vi "SS2 Live_Exit Cleanup.vi"(11 "SS2 Live Internal Variables":T1={"okCFrontPanelDevices Refnum"=refnum, "Device Refnum"=refnum, "Display Image"=refnum, "# Live Images"=0, "relative s"=0.0, "# Image Sets"=0, "Message"="", "Current Image Set"=0, "# Datasets"=0, "Current Dataset"=0, "Live Mode"=FALSE, "Recording Mode"=FALSE, "Record Button"=refnum, "Live Button"=refnum, "SS2 Live Gate Data Q Name"="", "Discard First Image"=FALSE, "Image Information"={"Save ROI Only"=FALSE, "Left"=0, "Top"=0, "Right"=0, "Bottom"=0, "Use Current ROI"=FALSE}, "Image Binning Options"={"Use Image Binning"=FALSE, "X Bin"=0, "Y Bin"=0}, "FPGA Serial Number"="", "PCB Version"=enum."PCB 1"} {"Image Binning Options"."Y Bin" min=1; "Image Binning Options"."X Bin" min=1}) -> ()   [LabVIEW 2019]
uses:
  SS2 Live Internal Variables.ctl
  C:/UCLA Thinkpad Google Drive/LabVIEW 2019 SP1/builds/SS2 Live Distribution/Opal Kelly/C# Wrapper/libFrontPanel-csharp.dll
  Opal Kelly/C# Wrapper/libFrontPanel-csharp.dll
  <vilib>/vision/Image Controls.llb/IMAQ Image.ctl
  SS2 Live_Image ROI Information.ctl
  Phasor/Image Binning Options.ctl
  SS2 DAQ PCB Version.ctl
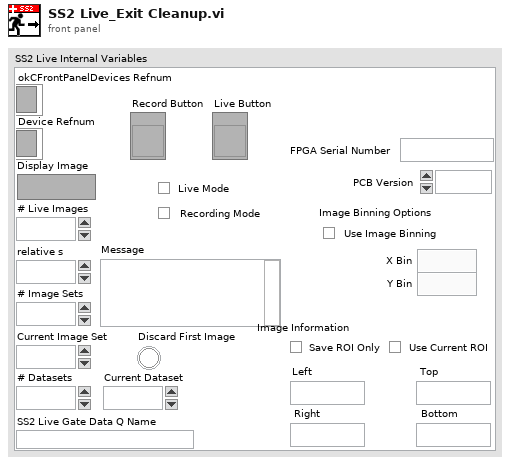
[diagram p1: front panel]
types:
  T1 = typedef "SS2 Live Internal Variables.ctl" = cluster{"okCFrontPanelDevices Refnum":refnum<k24>, "Device Refnum":refnum<k24>, "Display Image":T2, "# Live Images":i32, "relative s":dbl, "# Image Sets":i32, "Message":string, "Current Image Set":i32, "# Datasets":i32, "Current Dataset":i32, "Live Mode":bool, "Recording Mode":bool, "Record Button":refnum<vi>, "Live Button":refnum<vi>, "SS2 Live Gate Data Q Name":string, "Discard First Image":bool, "Image Information":T3, "Image Binning Options":T4, "FPGA Serial Number":string, "PCB Version":T5}
  T2 = typedef "IMAQ Image.ctl" = refnum<image>
  T3 = typedef "SS2 Live_Image ROI Information.ctl" = cluster{"Save ROI Only":bool, "Left":u16, "Top":u16, "Right":u16, "Bottom":u16, "Use Current ROI":bool}
  T4 = typedef "Image Binning Options.ctl" = cluster{"Use Image Binning":bool, "X Bin":i32, "Y Bin":i32}
  T5 = typedef "SS2 DAQ PCB Version.ctl" = enum16{"unknown", "PCB 1", "PCB 2"}
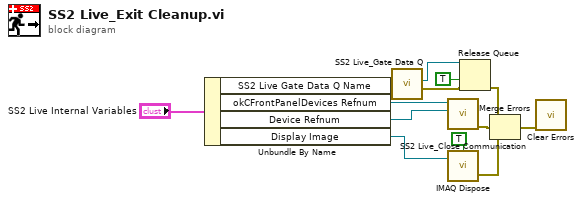
[diagram p0: block diagram]
diagram:
  n1 = Unbundle By Name("SS2 Live Internal Variables") -> ("SS2 Live Gate Data Q Name"=w11:string, "okCFrontPanelDevices Refnum"=w5:refnum<k24>, "Device Refnum"=w6:refnum<k24>, "Display Image"=w4:T2)
  n2 = call "SS2 Live_Gate Data Q.vi"("SS2 Live Gate Data Q Name"=w11) -> ("error out"=w12:errorcluster, "SS2 Live Gate Data Q"=w13:refnum<queue>)  [unwired: 5 in]
  n3 = call "SS2 Live_Close Communication.vi"("Device Refnum"=w6, "okCFrontPanelDevices Refnum"=w5) -> ("Error Out"=w7:errorcluster)  [unwired: 9 in]
  n4 = call "IMAQ Dispose"("All Images? (No)"=TRUE, "Image"=w4) -> ("error out"=w9:errorcluster)  [unwired: 4 in]
  n5 = Release Queue(queue=w13, force destroy? (F)=TRUE, error in (no error)=w12) -> (error out=w10:errorcluster)  [unwired: 2 out]
  n6 = Merge Errors(w10, w7, w9) -> (w8:errorcluster)
  n7 = call <vilib>:"Clear Errors.vi"("error in (no error)"=w8) -> ()  [unwired: 5 in, 2 out]
